vi "Add Monitor Status Channel.vi"(8 "error in (no error)":errorcluster, 11 "Section Ptr":T1 format="%.0x") -> (0 "error out":errorcluster, 3 "Parent Ref out":T1 format="%.0x")   [LabVIEW 2020, in "AIM ARINC 664 Scripting.lvlib"]
uses:
  AIM ARINC 664 Scripting.lvlib
  <vilib>/NI VeriStand/Custom Device API/Custom Device Item Ref.ctl
  <vilib>/NI VeriStand/Custom Device API/Custom Device Channel.ctl
  <vilib>/NI VeriStand/Custom Device API/Custom Device Channel Type.ctl
  Constants.vi
  <vilib>/NI VeriStand/Custom Device API/Custom Device API.lvlib
  <vilib>/Utility/Data Type/NI_Data Type.lvlib
  <vilib>/NI/NI VeriStand Advanced SysDef API/SysDef API/Advanced System Definition.lvlib
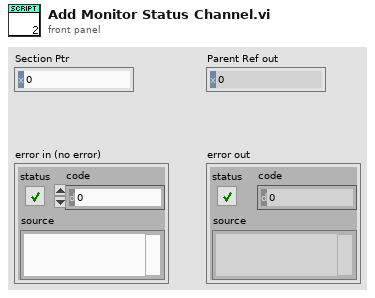
[diagram p1: front panel]
types:
  T1 = typedef "Custom Device API.lvlib/Custom Device Item Ref.ctl" = u64
  T2 = enum16{"FDX_MON_STAT_EMPTY", "FDX_MON_STAT_FILLED", "FDX_MON_STAT_FULL", "FDX_MON_STAT_OVERFLOW", "FDX_MON_STAT_ERROR"}
  T3 = typedef "Custom Device API.lvlib/Custom Device Channel.ctl" = cluster{"Type":T4, "Units":string, "Default Value":dbl, "Faultable":bool, "Scalable":bool}
  T4 = typedef "Custom Device API.lvlib/Custom Device Channel Type.ctl" = enum16{"Input", "Output"}
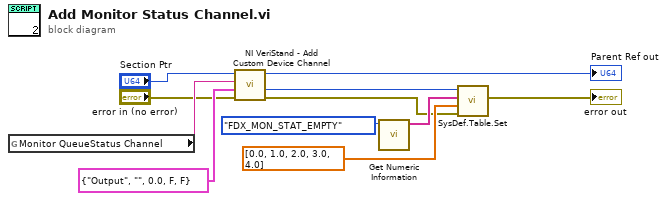
[diagram p0: block diagram]
diagram:
  n1 = global read "Constants.vi" "Monitor QueueStatus Channel"() -> (w3:string)
  n2 = call <vilib>:"NI VeriStand - Add Custom Device Channel.vi"("error in (no error)"="error in (no error)", "Channel"=T3 {"Type"=enum."Output", "Units"="", "Default Value"=0.0, "Faultable"=FALSE, "Scalable"=FALSE}, "Channel Name"=w3, "Parent Ref in"="Section Ptr") -> ("error out"=w5:errorcluster, "Channel Ref"=w7:T1, "Parent Ref out"=→"Parent Ref out":T1)  [unwired: 4 in, 1 out]
  n3 = call <vilib>:"Get Numeric Information.vi"("variant"=T2."FDX_MON_STAT_EMPTY" ("Enum")) -> ("enum names"=w8:string[])  [unwired: 7 in, 3 out]
  n4 = call <vilib>:"SysDef.Table.Set.vi"("error in (no error)"=w5, "Values"=dbl[] [0.0, 1.0, 2.0, 3.0, 4.0], "Names"=w8, "nodeID"=w7) -> ("error out"=→"error out":errorcluster)  [unwired: 6 in, 1 out]
